vi "Consumer.vi"(8 "error in (no error)":errorcluster, 9 "Data":variant, 10 "Case ID":string, 11 "uService Template in":refnum<class "Pizza Machine.lvclass">) -> (0 "error out":errorcluster, 3 "uService Template out":refnum<class "Pizza Machine.lvclass">)   [LabVIEW 2020, in "Pizza Machine.lvlib" / "Pizza Machine.lvclass"]
uses:
  Pizza Machine.lvclass
  Pizza Machine Consumer Case Selector.ctl
  Pizza Machine.lvclass/Pizza Machine.ctl
  TALOS/TALOS_PPL.lvlibp/Father of all uServices/Father of all uServices/Father of all uServices.lvclass
  TALOS/TALOS_PPL.lvlibp
  C:/LabVIEW Code/aegis-labview-code/TALOS/TALOS_PPL.lvlibp/Father of all uServices/Father of all uServices/Father of all uServices.lvclass
  C:/LabVIEW Code/aegis-labview-code/TALOS/TALOS_PPL.lvlibp/Ancestor/Ancestor/Ancestor.lvclass
  C:/LabVIEW Code/aegis-labview-code/TALOS/Actor Framework.lvlibp/1abvi3w/vi.lib/ActorFramework/Actor/Actor.lvclass
  C:/LabVIEW Code/aegis-labview-code/Other uServices/Pizza Machine/Pizza Machine.lvclass
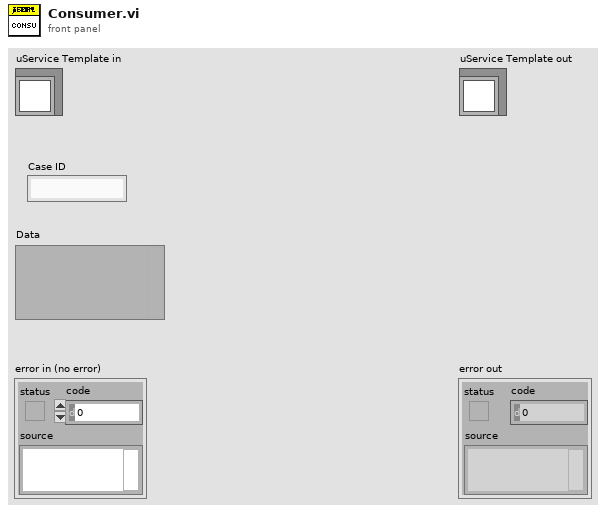
[diagram p1: front panel]
types:
  T1 = typedef "Pizza Machine.lvlib/Pizza Machine.lvclass/Pizza Machine Consumer Case Selector.ctl" = enum16{"Make Pizza"}
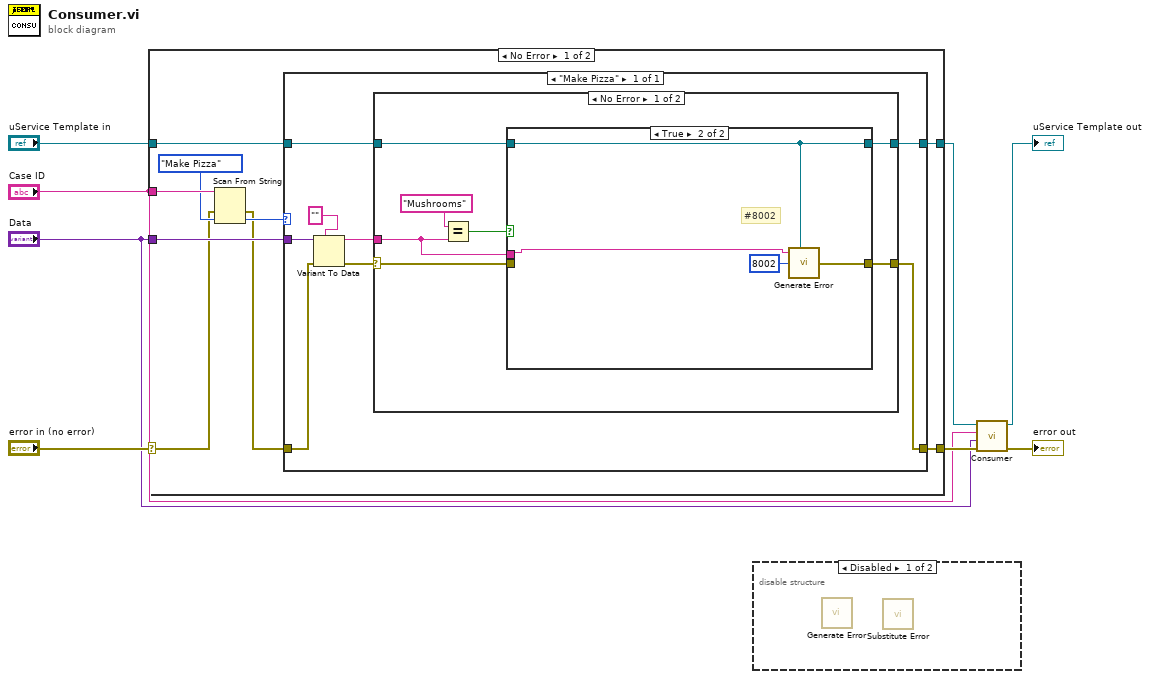
[diagram p0: block diagram]
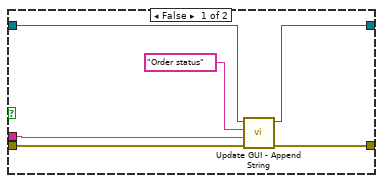
[diagram p3: hidden frame]
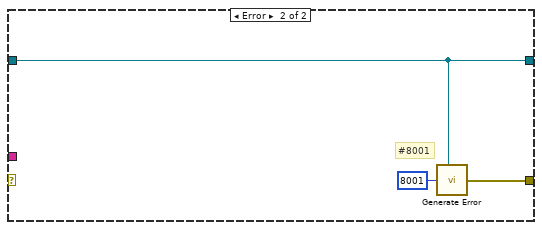
[diagram p4: hidden frame]
diagram:
  n1 = case shown="No Error" "error in (no error)" {
    selector: "error in (no error)" -> [w10 w46]
    tunnel: [w16 w47] -> w3
    tunnel: "uService Template in" -> [w17 w47]
    tunnel: [w14 w46] -> w6
    tunnel: "Case ID" -> [w13 _]
    tunnel: "Data" -> [w15 _]
    frame No Error {
      n2 = Scan From String(input string=w13, error in=w10, default 1=Pizza_Machine_Consumer_Case_Selector."Make Pizza" ("Consumer Case Selector")) -> (error out=w9:errorcluster, output 1=w11:T1)  [unwired: 2 in, 2 out]
      n3 = case shown="\"Make Pizza\"" w11 {
        tunnel: w17 -> [w23]
        tunnel: [w24] -> w16
        tunnel: w15 -> [w22]
        tunnel: [w25] -> w14
        tunnel: w9 -> [w21]
        frame "Make Pizza" {
          n4 = Variant To Data(error in=w21, type="", Variant=w22) -> (data=w19:string, error out=w20:errorcluster)
          n5 = case shown="No Error" w20 {
            selector: w20 -> [w32 _]
            tunnel: [w31 w45] -> w25
            tunnel: [w30 w44] -> w24
            tunnel: w23 -> [w29 w44]
            tunnel: w19 -> [w26 _]
            frame No Error {
              n6 = Equal?(x="Mushrooms", y=w26) -> (x = y?=w27:bool)
              n7 = case shown="True" w27 {
                tunnel: w32 -> [w38 _]
                tunnel: [w37 w41] -> w31
                tunnel: [w36 w42] -> w30
                tunnel: w29 -> [w35 w42]
                tunnel: w26 -> [w33 w39]
                frame False {
                  n8 = call "Update GUI - Append String.vi"("error in (no error)"=w38, "String"=w33, "GUI Item Name"="Order status", "Father of all uServices in"=w35) -> ("error out"=w37:errorcluster, "Father of all uServices out"=w36:refnum<class "Pizza Machine.lvclass">)  [unwired: 6 in]
                }
                frame True {
                  # "#8002"
                  n9 = call "Generate Error.vi"("Optional String"=w39, "Class"=w42, "Error Code"=8002) -> ("error out"=w41:errorcluster)  [unwired: 4 in]
                }
              }
            }
            frame Error {
              # "#8001"
              n10 = call "Generate Error.vi"("Class"=w44, "Error Code"=8001) -> ("error out"=w45:errorcluster)  [unwired: 5 in]
            }
          }
        }
      }
    }
    frame Error {
    }
  }
  n11 = disable-structure shown="Disabled" {
    frame Disabled {
      n12 = call "Generate Error.vi"() -> ()  [unwired: 7 in, 1 out]
      n13 = call "Substitute Error.vi"() -> ()  [unwired: 11 in, 1 out]
    }
    frame Enabled {
    }
  }
  n14 = call-parent "Consumer.vi"("error in (no error)"=w6, "Data"="Data", "Case ID"="Case ID", "uService Template in"=w3) -> ("error out"=→"error out":errorcluster, "uService Template out"=→"uService Template out":refnum<class "Pizza Machine.lvclass">)  [unwired: 6 in]
